vi "FinishFloatString.vi"(0 "Remove trailing zeroes?":bool, 5 "Precision":i16, 7 "String":string) -> (8 "Finished string":string)   [LabVIEW 2017, in "GPString.lvlib"]
doc: "Removes trailing zeroes from <B>String</B> if specified, and eliminates negative zero if necessary.\n\nThis VI is inlined.\n\nSteen Schmidt\nGPower\n25/9 2015"
uses:
  GPString.lvlib
panel:
  # "Copyright © 2015\nGPower\nSee enclosed license file for terms and conditions"
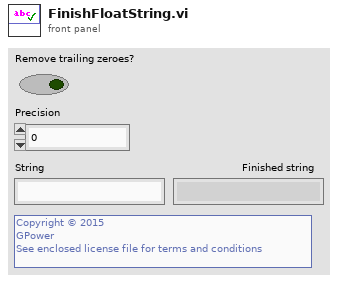
[diagram p1: front panel]
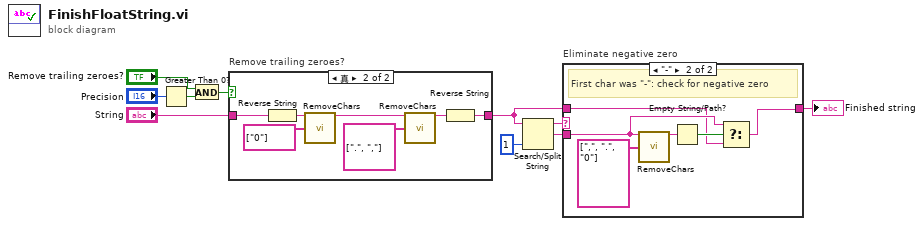
[diagram p0: block diagram]
diagram:
  n1 = Greater Than 0?(x="Precision") -> (x > 0?=w6:bool)
  n2 = And(x="Remove trailing zeroes?", y=w6) -> (x .and. y?=w2:bool)
  n3 = case "Remove trailing zeroes?" shown="真" w2 {
    tunnel: "String" -> [w11 w18]
    tunnel: [w11 w15] -> w9
    frame False {
    }
    frame True {
      n4 = Reverse String(1:w18) -> (0:w17:string)
      n5 = call "RemoveChars.vi"("String"=w17, "Chars to remove"=string[] ["0"]) -> ("Shortened string"=w13:string)  [unwired: 13 in]
      n6 = call "RemoveChars.vi"("String"=w13, "Chars to remove"=string[] [".", ","]) -> ("Shortened string"=w12:string)  [unwired: 13 in]
      n7 = Reverse String(1:w12) -> (0:w15:string)
    }
  }
  n8 = Search/Split String(string=w9, offset (0)=1) -> (substring before match=w8:string, match + rest of string=w10:string)  [unwired: 1 in, 1 out]
  n9 = case "Eliminate negative zero" shown="\"-\"" w8 {
    tunnel: w9 -> [w19 w21]
    tunnel: [w19 w20] -> w1
    tunnel: w10 -> [_ w22]
    frame Default {
      # "Can't be negative zero"
    }
    frame "-" {
      # "First char was \"-\": check for negative zero"
      n10 = call "RemoveChars.vi"("String"=w22, "Chars to remove"=string[] [",", ".", "0"]) -> ("Shortened string"=w24:string)  [unwired: 13 in]
      n11 = Empty String/Path?(string/path=w24) -> (empty?=w23:bool)
      n12 = Select(t=w22, s=w23, f=w21) -> (s? t:f=w20:string)
    }
  }
  "Finished string" <- w1
